vi "ALTS-2015 LV2GBL Error.vi"(9 "error in (no error)":errorcluster, 10 "Operation":enum16{"Init", "Set", "Get"}(ring)=enum."Set") -> (1 "error out":errorcluster)   [LabVIEW 2013]
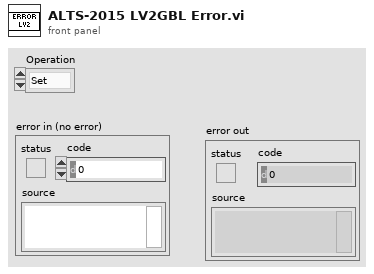
[diagram p1: front panel]
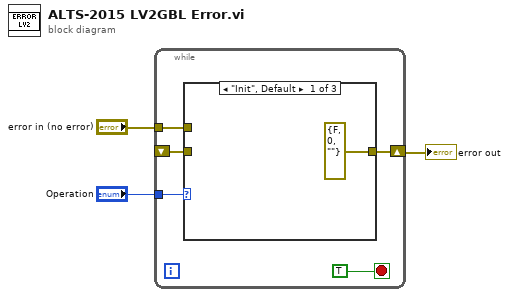
[diagram p0: block diagram]
diagram:
  n1 = while {
    shift-right: [w6] -> w3
    shift-left: _ -> [w7]
    tunnel: "Operation" -> [w5]
    tunnel: "error in (no error)" -> [w4]
    stop <- TRUE stop-if-true
    n2 = case shown="\"Init\", Default" w5 {
      tunnel: w7 -> [_ _ w11]
      tunnel: [errorcluster {"status"=FALSE, "code"=0, "source"=""} ("error in (no error)") w10 w11] -> w6
      tunnel: w4 -> [_ w10 _]
      frame "Init", Default {
      }
      frame "Set" {
      }
      frame "Get" {
      }
    }
  }
  "error out" <- w3
